vi "Fullspec (SubVI).vi"(0 "Compensate SR":bool, 1 "revolutions to display [rev]":cluster{"start":dbl, "duration":dbl}={"start"=0.0, "duration"=1.0} {"duration" format="%.2f"; "start" format="%.2f"}, 2 "shaft rotating direction":u16(ring) items=["CCW", "CW"], 5 "Reset SR":bool, 7 "AutSR":dbl, 9 "Sensors":waveform(dbl)[](array[waveform]), 10 "threshold (auto)":dbl=inf, 11 "error in (no error)":errorcluster, 12 "probe angle X [deg]":u16=45, 13 "probe angle Y [deg]":u16=135, 14 "window":u32(ring)=1 items=["None"=0, "Hanning"=1, "Hamming"=2, "Blackman-Harris"=3, "Exact Blackman"=4, "Blackman"=5, "Flat Top"=6, "4 Term B-Harris"=7, "7 Term B-Harris"=8, "Low Sidelobe"=9, "Gaussian"=62]) -> (3 "Execute  MATSCRIPT":bool, 4 "orbit/timebase plot":T1(array[cluster]), 6 "Full Spectrum":T2(graph)={"order 0"=-44.0, "delta order"=0.0859375, "magnitude"=[]}, 8 "even-angle references":cluster{"r0":dbl, "dr":dbl, "Y":dbl[]}[](array[cluster]), 15 "error out":errorcluster)   [LabVIEW 2012]
uses:
  <vilib>/Waveform/WDTOps.llb/WDT Index Channel DBL.vi
  <vilib>/Analysis/baseanly.llb/Mean (DBL).vi
  <vilib>/addons/Sound and Vibration/Order Analysis/Tach Process/OAT Analog Tacho Process (1 Tacho).vi
  <vilib>/addons/Sound and Vibration/Order Analysis/Resample Order Tracking/OAT Convert to Even Angle Signal (N Channels).vi
  <vilib>/addons/Sound and Vibration/Order Analysis/Referece Data Processing/OAT Get Even Angle Reference (N Channels).vi
  <vilib>/addons/Sound and Vibration/Order Analysis/Referece Data Processing/OAT Compensate Even Angle Signal (Even Angle Ref, N Channels).vi
  <vilib>/addons/Sound and Vibration/Order Analysis/Data Presentation/SVX Orbit and Timebase Plot (Unfiltered).vi
  <vilib>/addons/Sound and Vibration/Order Analysis/Tach Process/SoundVib_TachProcess.lvlib
  <vilib>/addons/Sound and Vibration/Order Analysis/Resample Order Tracking/SoundVib_OrderTracking.lvlib
  <vilib>/Analysis/NI_AALBase.lvlib
  <vilib>/addons/Sound and Vibration/Order Analysis/Referece Data Processing/SoundVib_RefDataProcess.lvlib
  <vilib>/addons/Sound and Vibration/Order Analysis/Data Presentation/SoundVib_MCMDisplay.lvlib
panel:
  out "error out 3":errorcluster
  out "error out 2":errorcluster
  out "even-angle ref aux":cluster{"r0":dbl, "dr":dbl, "Y":dbl[]}[](array[cluster])
  out "error out 5":errorcluster
  out "error out 4":errorcluster
  out "Waveform Graph 4":cluster{"r0":dbl, "dr":dbl, "Y":dbl[]}[](graph)
  out "Waveform Graph":cluster{"r0":dbl, "dr":dbl, "Y":dbl[]}[](graph)
  out "Waveform Graph 2":waveform(dbl)[](graph)
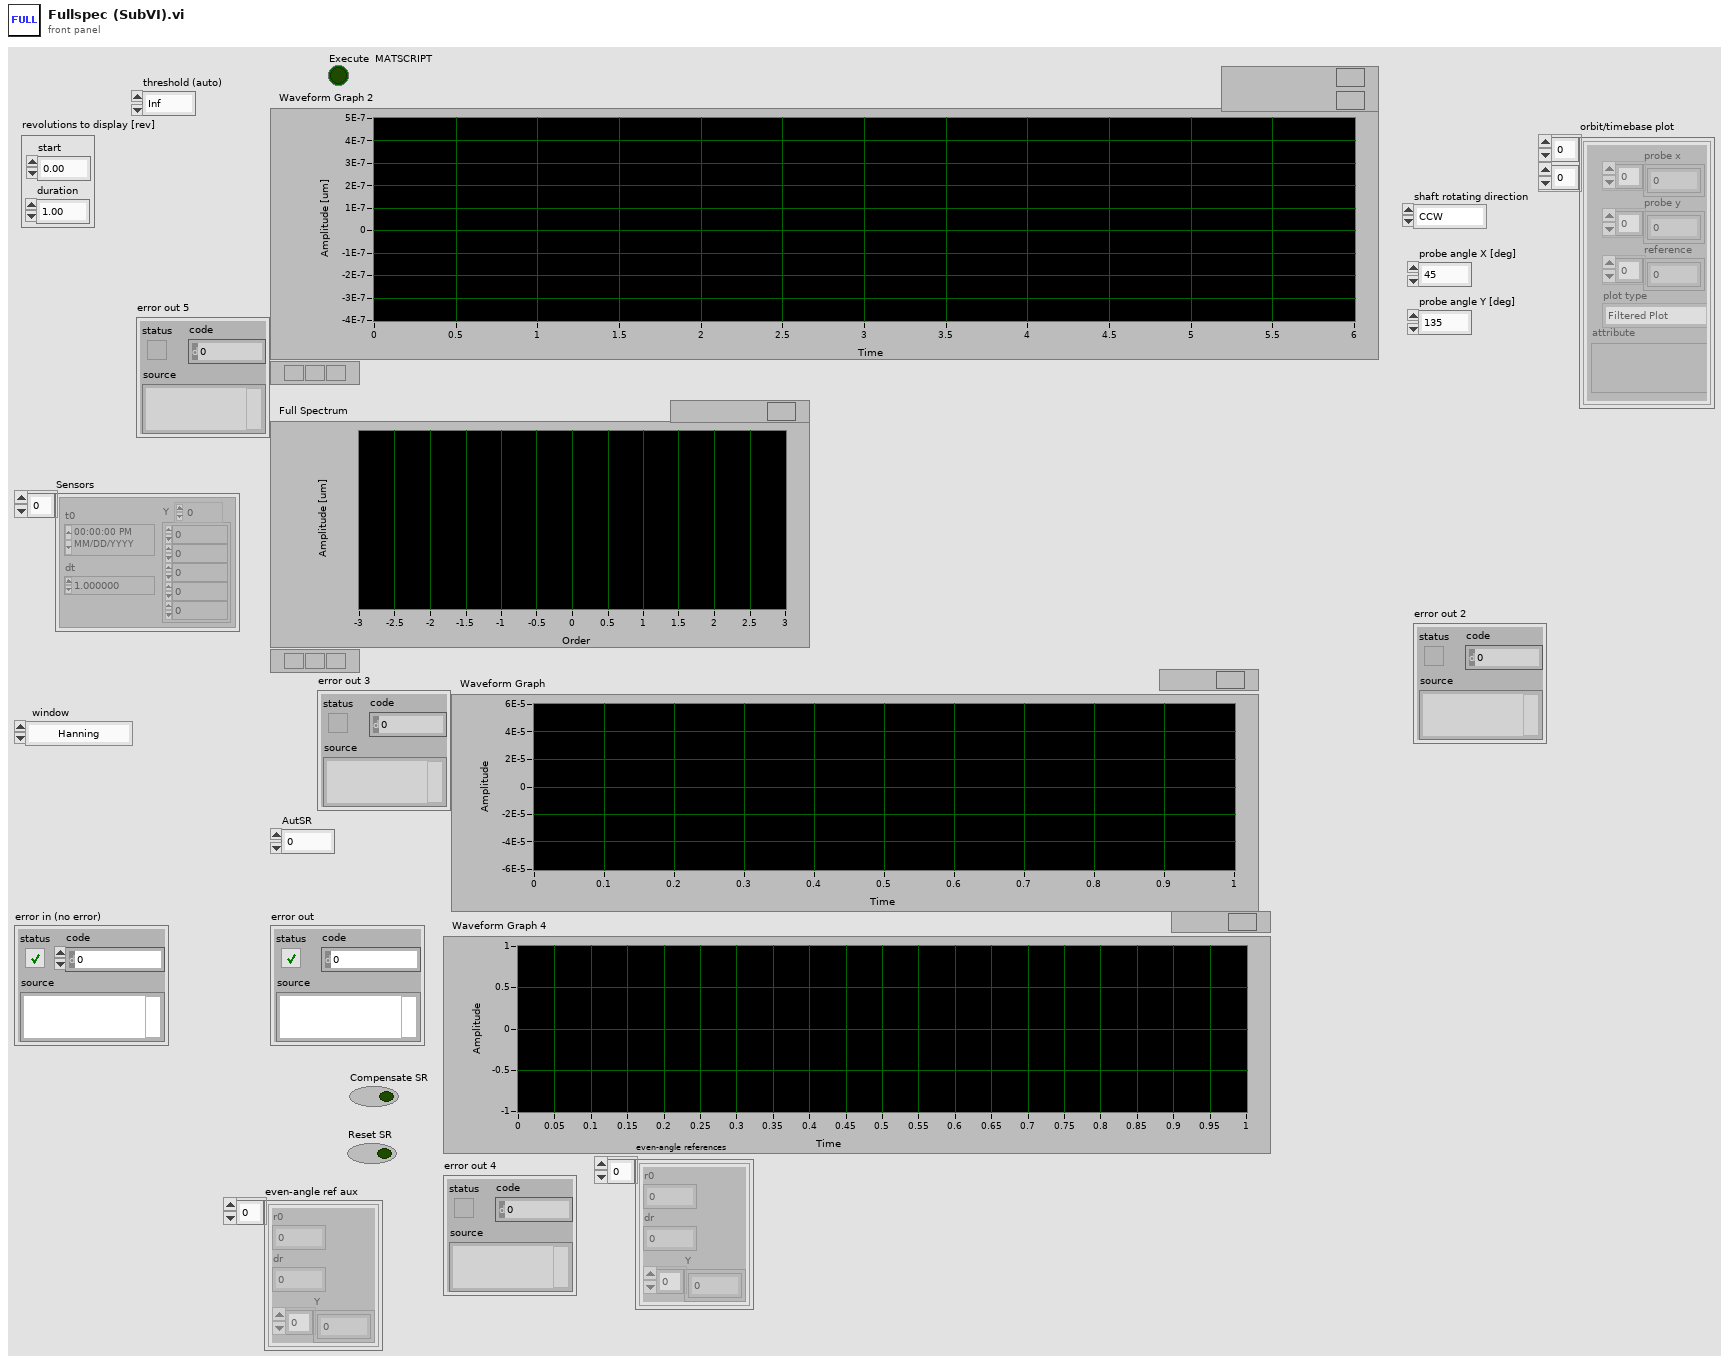
[diagram p1: front panel]
types:
  T1 = cluster{"probe x":dbl[], "probe y":dbl[], "reference":dbl[], "plot type":enum16{"Filtered Plot", "Unfiltered Plot"}, "attribute":variant}[][]
  T2 = cluster{"order 0":dbl, "delta order":dbl, "magnitude":dbl[]}
  T3 = typedef "SoundVib_TachProcess.lvlib/speed profile.ctl" = cluster{"time [s]":dbl[], "speed [RPM]":dbl[]}
  T4 = typedef "svc_Resampled Channel Info.ctl" = cluster{"channel name":string, "description":string, " channel info":T5}
  T5 = typedef "svc_Channel Info.ctl" = cluster{"sensor sensitivity [mV/EU]":dbl, "engineering units":T6, "dB reference [EU]":dbl, "custom label":string, "weighting filter":T7, "pregain [dB]":dbl}
  T6 = typedef "svc_Engineering Units Text Ring.ctl" = u16
  T7 = typedef "svc_Weighting Filter Text Ring.ctl" = u16
  T8 = typedef "OAT Position Info.ctl" = cluster{"positions [s]":dbl[], "samples/rev":dbl}
  T9 = typedef "svl_Resampled Channel Info.ctl" = cluster{"channel name":string, "description":string, " channel info":T10}
  T10 = typedef "svl_Channel Info.ctl" = cluster{"sensor sensitivity [mV/EU]":dbl, "engineering units":T11, "dB reference [EU]":dbl, "custom label":string, "weighting filter":T12, "pregain [dB]":dbl}
  T11 = typedef "svl_Engineering Units Text Ring.ctl" = u16
  T12 = typedef "svl_Weighting Filter Text Ring.ctl" = u16
  T13 = cluster{"shaft rotating direction":u16, "probe angle X [deg]":u16, "element":u16}
  T14 = cluster{"shaft rotating direction":u16, "probe angle Y [deg]":u16, "element":u16}
  T15 = cluster{"shaft rotating direction":u16, "probe angle Y [deg]":u16, "element":u16}[]
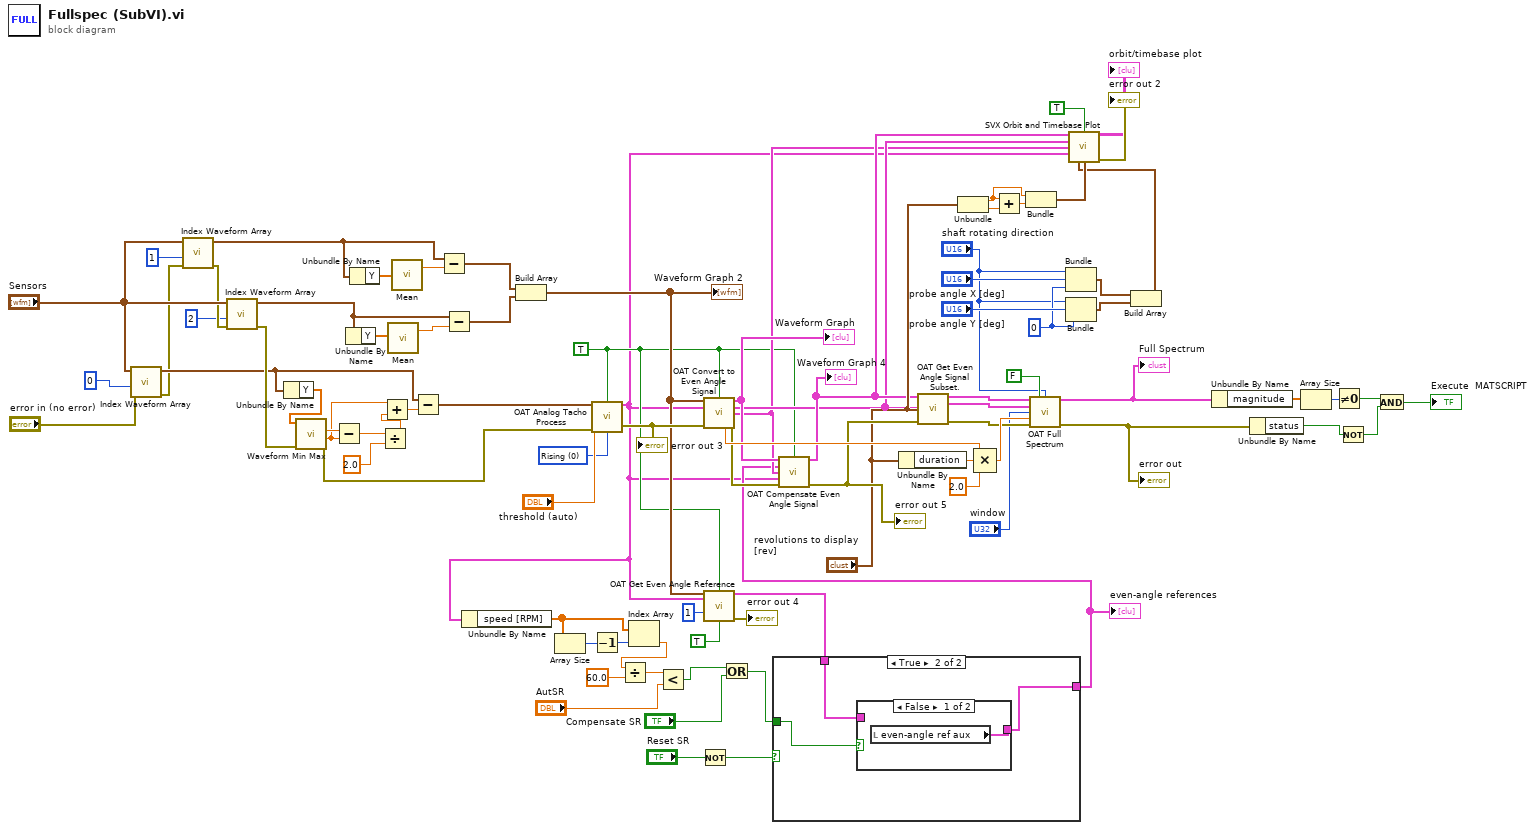
[diagram p0: block diagram]
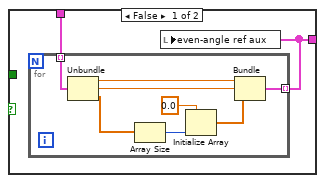
[diagram p2: hidden frame]
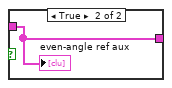
[diagram p3: hidden frame]
diagram:
  w22 = u16 0 ("element")
  w25 = TRUE ("reset? (F)")
  w77 = u16 0 items=["Rising", "Falling"] ("slope (Rising)")
  n1 = call-poly <vilib>:"Index Waveform Array.vi"("error in (no error)"="error in (no error)", "index"=0, "waveform array"="Sensors") -> ("error out"=w57:errorcluster, "waveform"=w76:waveform(dbl))  [unwired: 7 in]
  n2 = call-poly <vilib>:"Index Waveform Array.vi"("error in (no error)"=w57, "index"=1, "waveform array"="Sensors") -> ("error out"=w56:errorcluster, "waveform"=w16:waveform(dbl))  [unwired: 7 in]
  n3 = call-poly <vilib>:"Index Waveform Array.vi"("error in (no error)"=w56, "index"=2, "waveform array"="Sensors") -> ("error out"=w80:errorcluster, "waveform"=w86:waveform(dbl))  [unwired: 7 in]
  n4 = Unbundle By Name(w76) -> ("Y"=w75:dbl[])
  n5 = call <vilib>:"Waveform Min Max.vi"("error in (no error)"=w80, "waveform in"=w75) -> ("error out"=w79:errorcluster, "Y min"=w74:dbl, "Y max"=w84:dbl)  [unwired: 4 in, 3 out]
  n6 = Subtract(x=w84, y=w74) -> (x-y=w83:dbl)
  n7 = Unbundle By Name(w86) -> ("Y"=w62:dbl[])
  n8 = Unbundle By Name(w16) -> ("Y"=w60:dbl[])
  n9 = Divide(x=w83, y=2.0) -> (x/y=w73:dbl)
  n10 = Add(x=w74, y=w73) -> (x+y=w72:dbl)
  n11 = call-poly <vilib>:"Mean.vi"("X"=w62) -> ("mean"=w61:dbl)  [unwired: 1 out]
  n12 = call-poly <vilib>:"Mean.vi"("X"=w60) -> ("mean"=w59:dbl)  [unwired: 1 out]
  n13 = Subtract(x=w76, y=w72) -> (x-y=w45:waveform(dbl))
  n14 = Subtract(x=w16, y=w59) -> (x-y=w12:waveform(dbl))
  n15 = Subtract(x=w86, y=w61) -> (x-y=w63:waveform(dbl))
  n16 = Build Array(w12, w63) -> (w38:waveform(dbl)[])
  "Waveform Graph 2" <- w38
  n17 = call-poly <vilib>:"OAT Analog Tacho Process.vi"("analog tacho signal"=w45, "reset? (F)"=w25, "threshold (auto)"="threshold (auto)", "error in (no error)"=w79, "slope (Rising)"=w77) -> ("speed profile"=w11:T3, "error out"=w87:errorcluster)  [unwired: 6 in, 3 out]
  "error out 3" <- w87
  n18 = Unbundle By Name(w11) -> ("speed [RPM]"=w9:dbl[])
  n19 = Array Size(array=w9) -> (size(s)=w8:i32)
  n20 = Decrement(x=w8) -> (x-1=w7:i32)
  n21 = Index Array(array=w9, index=w7) -> (element=w6:dbl)
  n22 = Divide(x=w6, y=60.0) -> (x/y=w10:dbl)
  n23 = Less?(x=w10, y="AutSR") -> (x < y?=w4:bool)
  n24 = Not(x="Reset SR") -> (.not. x?=w37:bool)
  n25 = call-poly <vilib>:"OAT Convert to Even Angle Signal.vi"("scaled signals [EU]"=w38, "reset? (F)"=w25, "speed profile"=w11, "error in (no error)"=w87) -> ("even-angle signals"=w44:cluster{"r0":dbl, "dr":dbl, "Y":dbl[]}[], "even-angle channel info"=w28:T4[], "even-angle position info"=w27:T8, "actual max order"=w68:dbl, "error out"=w43:errorcluster)  [unwired: 3 in, 4 out]
  "Waveform Graph" <- w44
  n26 = call-poly <vilib>:"OAT Get Even Angle Reference.vi"("scaled signals [EU]"=w38, "reset? (F)"=w25, "speed profile"=w11, "# of revs in reference"=1, "remove DC? (F)"=TRUE) -> ("even-angle references"=w14:cluster{"r0":dbl, "dr":dbl, "Y":dbl[]}[], "error out"=→"error out 4":errorcluster)  [unwired: 8 in, 1 out]
  n27 = Or(x=w4, y="Compensate SR") -> (x .or. y?=w2:bool)
  n28 = case shown="True" w37 {
    tunnel: [w89 w100] -> w13
    tunnel: w2 -> [_ w99]
    tunnel: w14 -> [w88 w98]
    frame False {
      n29 = for {
        tunnel: [w95] -> w89 mode=indexing
        tunnel: w88 -> [w90] mode=indexing
        n30 = Unbundle(w90) -> ("r0"=w97:dbl, "dr"=w96:dbl, "Y"=w94:dbl[])
        n31 = Array Size(array=w94) -> (size(s)=w93:i32)
        n32 = Initialize Array(0.0 ("element"), w93) -> (w91:dbl[])
        n33 = Bundle("r0"=w97, "dr"=w96, w91) -> (w95:cluster{"r0":dbl, "dr":dbl, dbl[]})  [unwired: 1 out]
      }
      n34 = local write "even-angle ref aux"(w89) -> ()
    }
    frame True {
      n35 = case shown="False" w99 {
        tunnel: [w101 w102] -> w100
        tunnel: w98 -> [_ w102]
        frame False {
          n36 = local read "even-angle ref aux"() -> (w101:cluster{"r0":dbl, "dr":dbl, "Y":dbl[]}[])
        }
        frame True {
          "even-angle ref aux" <- w102
        }
      }
    }
  }
  "even-angle references" <- w13
  n37 = call-poly <vilib>:"OAT Compensate Even Angle Signal.vi"("even-angle signals"=w44, "reset? (F)"=w25, "even-angle references"=w13, "even-angle position info"=w27, "speed profile"=w11, "error in (no error)"=w43) -> ("compensated even-angle signals"=w29:cluster{"r0":dbl, "dr":dbl, "Y":dbl[]}[], "error out"=w42:errorcluster)  [unwired: 6 in, 2 out]
  "Waveform Graph 4" <- w29
  "error out 5" <- w42
  n38 = Unbundle By Name("revolutions to display [rev]") -> ("duration"=w69:dbl)
  n39 = call "OAT Get Even Angle Signal Subset..vi"("even angle signals (x-y)"=w29, "even angle channel info"=w28, "revolution subset [rev]"="revolutions to display [rev]", "error in (no error)"=w42) -> ("even angle signals (x-y) out"=w15:cluster{"r0":dbl, "dr":dbl, "Y":dbl[]}[], "dup even angle channel info"=w67:T9[], "error out"=w66:errorcluster)  [unwired: 9 out]
  n40 = Unbundle("revolutions to display [rev]") -> ("start"=w33:dbl, "duration"=w35:dbl)
  n41 = Compound Arithmetic op=MULTIPLY(w68, w69, 2.0 ("value")) -> (w71:dbl)
  n42 = Add(x=w33, y=w35) -> (x+y=w34:dbl)
  n43 = Bundle("start"=w33, w34) -> (w32:cluster{"start":dbl, dbl})  [unwired: 1 out]
  n44 = call "OAT Full Spectrum.vi"("even angle signals (x-y)"=w15, "dB on (T)"=FALSE, "shaft rotating direction"="shaft rotating direction", "even angle channel info"=w67, "window"="window", "block size"=w71, "error in (no error)"=w66) -> ("full spectrum"=w48:T2, "error out"=w47:errorcluster)  [unwired: 2 in, 5 out]
  "error out" <- w47
  "Full Spectrum" <- w48
  n45 = Bundle("shaft rotating direction"="shaft rotating direction", "probe angle X [deg]"="probe angle X [deg]", "element"=w22) -> (w21:T13)  [unwired: 1 in]
  n46 = Bundle("shaft rotating direction"="shaft rotating direction", "probe angle Y [deg]"="probe angle Y [deg]", "element"=w22) -> (w20:T14)  [unwired: 1 in]
  n47 = Build Array(w21, w20) -> (w18:T15)
  n48 = call-poly <vilib>:"SVX Orbit and Timebase Plot.vi"("even-angle signals"=w29, "reset? (F)"=TRUE, "even-angle channel info"=w28, "even-angle position info"=w27, "speed profile"=w11, "channel properties"=w18, "segment settings"=w32) -> ("orbit/timebase plot"=→"orbit/timebase plot":T1, "error out"=→"error out 2":errorcluster)  [unwired: 1 in, 6 out]
  n49 = Unbundle By Name(w48) -> ("magnitude"=w52:dbl[])
  n50 = Unbundle By Name(w47) -> ("status"=w49:bool)
  n51 = Array Size(array=w52) -> (size(s)=w53:i32)
  n52 = Not Equal To 0?(x=w53) -> (x != 0?=w51:bool)
  n53 = Not(x=w49) -> (.not. x?=w50:bool)
  n54 = And(x=w51, y=w50) -> (x .and. y?=→"Execute  MATSCRIPT":bool)
